vi "pressure caliberation.vi"() -> ()   [LabVIEW 2018]
uses:
  <vilib>/ptbypt/NI_PtbyPt.lvlib
panel:
  out "Actual Pressure in the muscle 12":dbl(knob) scale=0.0..30.0
  out "Actual Pressure in the muscle 11":dbl(knob) scale=0.0..30.0
  out "Actual Pressure in the muscle 6":dbl(knob) scale=0.0..30.0
  out "Actual Pressure in the muscle 7":dbl(knob) scale=0.0..30.0
  out "Actual Pressure in the muscle 2":dbl(knob) scale=0.0..30.0
  out "Actual Pressure in the muscle 4":dbl(knob) scale=0.0..30.0
  out "Actual Pressure in the muscle 1":dbl(knob) scale=0.0..30.0
  in  "stop (F) 3":bool caption="stop (F)"
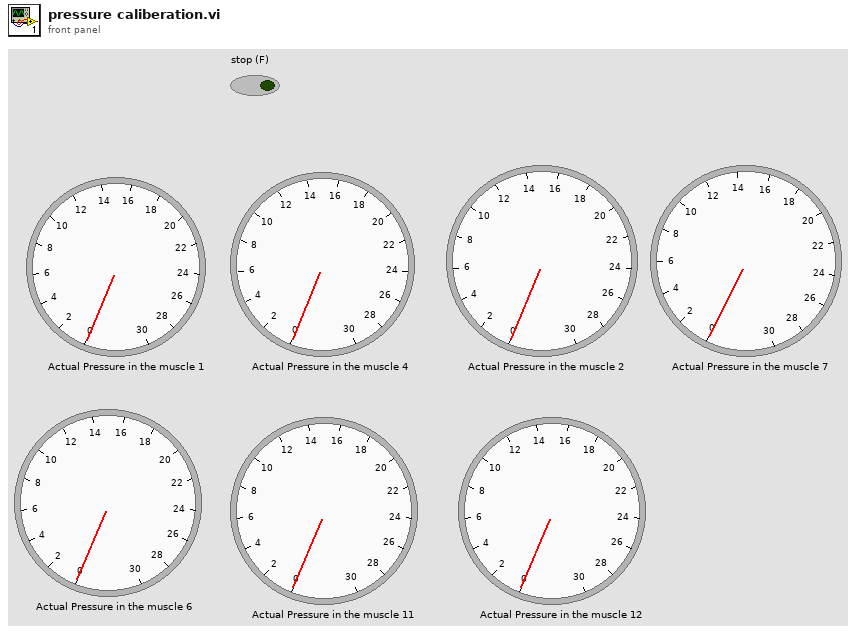
[diagram p1: front panel]
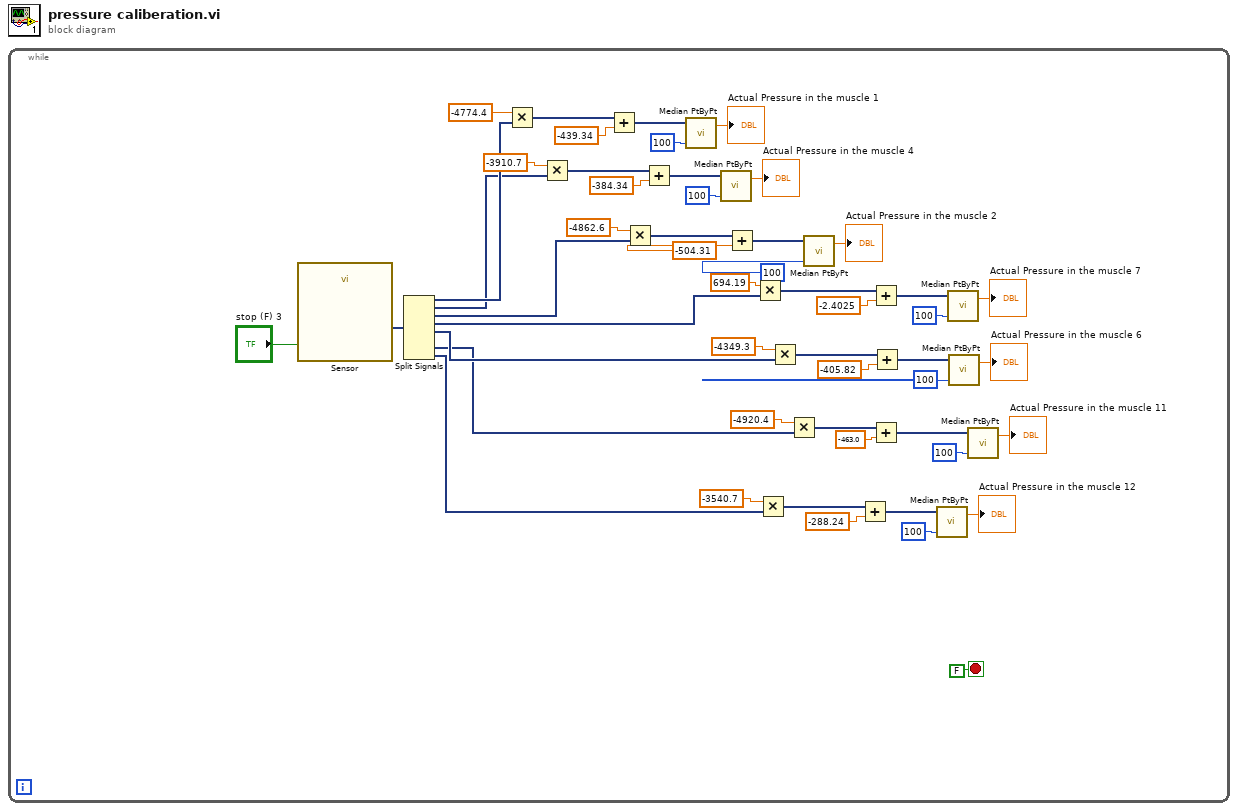
[diagram p0: block diagram]
diagram:
  n1 = while {
    stop <- FALSE stop-if-true
    n2 = call "Sensor"("stop (T)"="stop (F) 3") -> ("data"=w50:dynamicdata)  [unwired: 16 in, 2 out]
    n3 = Split Signals(w50) -> (w49:dynamicdata, w36:dynamicdata, w29:dynamicdata, w22:dynamicdata, w15:dynamicdata, w8:dynamicdata, w1:dynamicdata)  [unwired: 8 in, 1 out]
    n4 = Multiply(x=-4774.4, y=w49) -> (x*y=w52:dynamicdata)
    n5 = Multiply(x=-3910.7, y=w36) -> (x*y=w42:dynamicdata)
    n6 = Add(x=w52, y=-439.34) -> (x+y=w45:dynamicdata)
    n7 = Multiply(x=-4862.6, y=w29) -> (x*y=w35:dynamicdata)
    n8 = Add(x=w42, y=-384.34) -> (x+y=w39:dynamicdata)
    n9 = call <vilib>:"Median PtByPt.vi"("sample length"=100, "x"=w45) -> ("median"=→"Actual Pressure in the muscle 1":dbl)  [unwired: 2 in, 1 out]
    n10 = call <vilib>:"Median PtByPt.vi"("sample length"=100, "x"=w39) -> ("median"=→"Actual Pressure in the muscle 4":dbl)  [unwired: 2 in, 1 out]
    n11 = Add(x=w35, y=-504.31) -> (x+y=w32:dynamicdata)
    n12 = Multiply(x=694.19, y=w22) -> (x*y=w28:dynamicdata)
    n13 = Multiply(x=-3540.7, y=w1) -> (x*y=w7:dynamicdata)
    n14 = Multiply(x=-4349.3, y=w15) -> (x*y=w21:dynamicdata)
    n15 = Multiply(x=-4920.4, y=w8) -> (x*y=w14:dynamicdata)
    n16 = call <vilib>:"Median PtByPt.vi"("sample length"=100, "x"=w32) -> ("median"=→"Actual Pressure in the muscle 2":dbl)  [unwired: 2 in, 1 out]
    n17 = Add(x=w7, y=-288.24) -> (x+y=w4:dynamicdata)
    n18 = Add(x=w28, y=-2.4025) -> (x+y=w25:dynamicdata)
    n19 = Add(x=w14, y=-463.0) -> (x+y=w11:dynamicdata)
    n20 = Add(x=w21, y=-405.82) -> (x+y=w18:dynamicdata)
    n21 = call <vilib>:"Median PtByPt.vi"("sample length"=100, "x"=w4) -> ("median"=→"Actual Pressure in the muscle 12":dbl)  [unwired: 2 in, 1 out]
    n22 = call <vilib>:"Median PtByPt.vi"("sample length"=100, "x"=w25) -> ("median"=→"Actual Pressure in the muscle 7":dbl)  [unwired: 2 in, 1 out]
    n23 = call <vilib>:"Median PtByPt.vi"("sample length"=100, "x"=w18) -> ("median"=→"Actual Pressure in the muscle 6":dbl)  [unwired: 2 in, 1 out]
    n24 = call <vilib>:"Median PtByPt.vi"("sample length"=100, "x"=w11) -> ("median"=→"Actual Pressure in the muscle 11":dbl)  [unwired: 2 in, 1 out]
  }
